vi "YL get sn.vi"(8 "error in (no error)":errorcluster caption="错误输入（无错误）", 10 "探头型号":u16(ring) items=["电导率"=1, "DO"=2, "叶绿素a"=3, "pH"=4, "浊度"=20], 11 "MB session in":refnum<class "MB_Master.lvclass">) -> (0 "error out":errorcluster caption="错误输出", 2 "SN":string, 3 "MB session out":refnum<class "MB_Master.lvclass">)   [LabVIEW 2016, in "斯坦道多参数.lvlib"]
uses:
  <vilib>/Plasmionique/MB Master/MB_Master/MB_Master.lvclass
  <vilib>/Plasmionique/MB Master/MB Master.lvlib
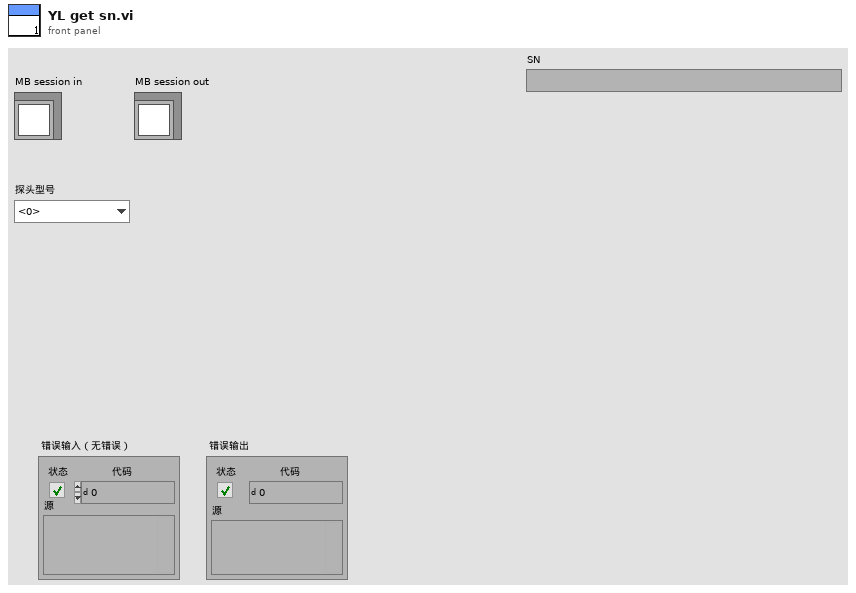
[diagram p1: front panel]
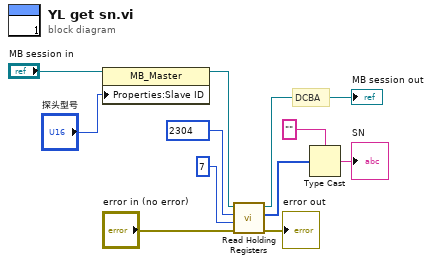
[diagram p0: block diagram]
diagram:
  # "DCBA"
  n1 = property class="MB_Master"(reference="MB session in", "Properties:Slave ID"="探头型号") -> (reference out=w8:refnum<class "MB_Master.lvclass">)  [unwired: 1 in, 1 out]
  n2 = call <vilib>:"Read Holding Registers.vi"("error in (no error)"="error in (no error)", "quantity"=u16 7, "starting address"=u16 2304, "MB session in"=w8) -> ("error out"=→"error out":errorcluster, "Registers"=w3:u16[], "MB session out"=→"MB session out":refnum<class "MB_Master.lvclass">)  [unwired: 5 in]
  n3 = Type Cast(type="", x=w3) -> (*(type *) &x=→"SN":string)
